vi "Zoom(User Event).vi"(8 "error in (no error)":errorcluster, 10 "Zoom":bool, 11 "XYGraphOverview in":refnum<class "XYGraphOverview.lvclass">) -> (0 "error out":errorcluster, 3 "XYGraphOverview out":refnum<class "XYGraphOverview.lvclass">)   [LabVIEW 2020, in "XYGraphOverview.lvlib" / "XYGraphOverview.lvclass"]
uses:
  XYGraphOverview.lvclass
  XYGraphOverview.lvclass/XYGraphOverview.ctl
  Read Block Color.vi
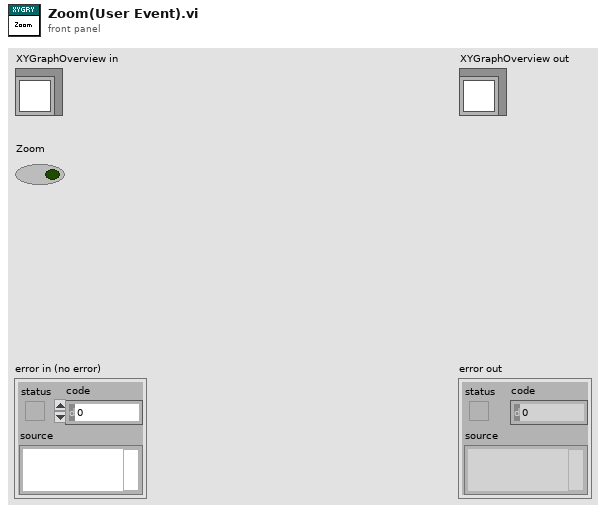
[diagram p1: front panel]
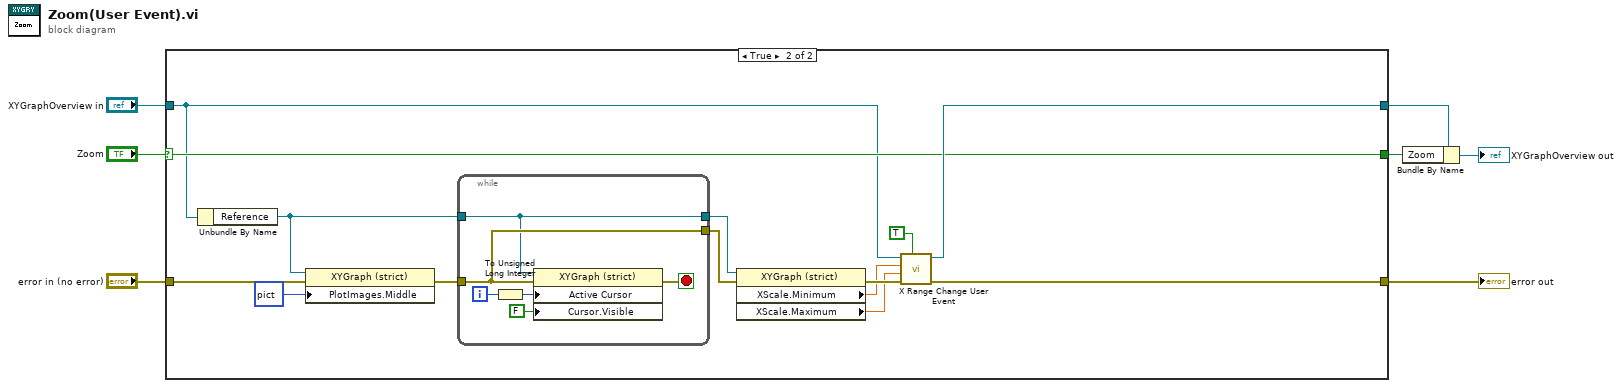
[diagram p0: block diagram]
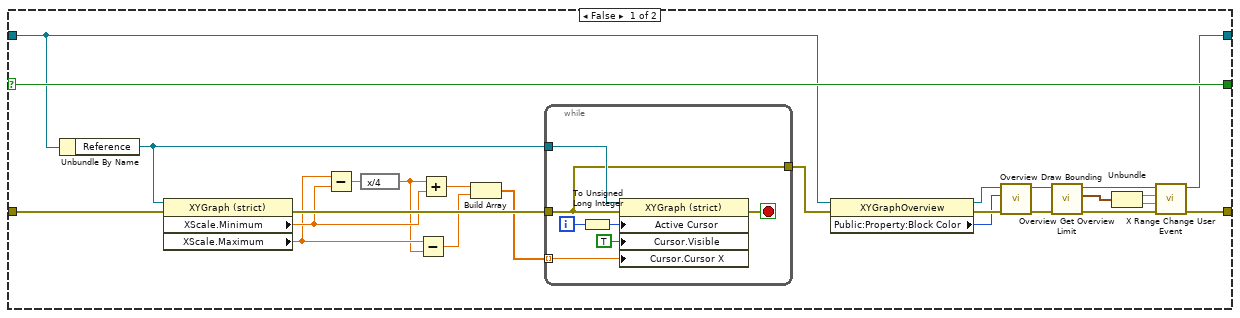
[diagram p2: hidden frame]
diagram:
  n1 = case shown="True" "Zoom" {
    selector: "Zoom" -> [w22 w46]
    tunnel: "error in (no error)" -> [w32 w52]
    tunnel: "XYGraphOverview in" -> [w9 w44]
    tunnel: [w8 w47] -> w3
    tunnel: [w10 w49] -> w7
    tunnel: [w22 w46] -> w2
    frame False {
      n2 = Unbundle By Name(w9) -> ("Reference"=w30:refnum<vi>)
      n3 = property class="XYGraph (strict)"(reference=w30, error in=w32) -> (error out=w31:errorcluster, "XScale.Minimum"=w28:dbl, "XScale.Maximum"=w27:dbl)  [unwired: 1 out]
      n4 = Subtract(x=w27, y=w28) -> (x-y=w29:dbl)
      n5 = expression code="x/4"(w29) -> (w26:dbl)
      n6 = Subtract(x=w27, y=w26) -> (x-y=w24:dbl)
      n7 = Add(x=w26, y=w28) -> (x+y=w25:dbl)
      n8 = Build Array(w25, w24) -> (w23:dbl[])
      n9 = while {
        tunnel: w31 -> [w34]
        tunnel: w30 -> [w35]
        tunnel: [w34] -> w11
        tunnel: w23 -> [w33] mode=indexing
        i -> [w38]
        stop <- w36 stop-if-true
        n10 = To Unsigned Long Integer(number=w38) -> (unsigned 32bit integer=w37:u32)
        n11 = property on="Property Node" class="XYGraph (strict)"(reference=w35, error in=w34, "Active Cursor"=w37, "Cursor.Visible"=TRUE, "Cursor.Cursor X"=w33) -> (error out=w36:errorcluster)  [unwired: 1 out]
      }
      n12 = property class="XYGraphOverview"(reference=w9, error in=w11) -> (reference out=w13:refnum<class "XYGraphOverview.lvclass">, error out=w14:errorcluster, "Public:Property:Block Color"=w12:u32)
      n13 = call "Overview Draw Bounding.vi"("error in (no error)"=w14, "Color"=w12, "XYGraphOverview in"=w13) -> ("error out"=w21:errorcluster, "XYGraphOverview out"=w20:refnum<class "XYGraphOverview.lvclass">)  [unwired: 7 in]
      n14 = call "Overview Get Overview Limit.vi"("error in"=w21, "XYGraphOverview in"=w20) -> ("error out"=w17:errorcluster, "Limit"=w19:cluster{"Lower Limit":dbl, "Upper Limit":dbl}, "XYGraphOverview out"=w18:refnum<class "XYGraphOverview.lvclass">)  [unwired: 7 in]
      n15 = Unbundle(w19) -> ("Lower Limit"=w16:dbl, "Upper Limit"=w15:dbl)
      n16 = call "X Range Change User Event.vi"("error in (no error)"=w17, "Upper Range"=w15, "Lower Range"=w16, "XYGraphOverview in"=w18) -> ("error out"=w10:errorcluster, "XYGraphOverview out"=w8:refnum<class "XYGraphOverview.lvclass">)  [unwired: 6 in]
    }
    frame True {
      n17 = Unbundle By Name(w44) -> ("Reference"=w50:refnum<vi>)
      n18 = property on="Property Node" class="XYGraph (strict)"(reference=w50, error in=w52, "PlotImages.Middle"=picture data[5B] ("Plot Images:Middle")) -> (error out=w51:errorcluster)  [unwired: 1 out]
      n19 = while {
        tunnel: w51 -> [w55]
        tunnel: w50 -> [w54]
        tunnel: [w55] -> w40
        tunnel: [w54] -> w45
        i -> [w58]
        stop <- w56 stop-if-true
        n20 = To Unsigned Long Integer(number=w58) -> (unsigned 32bit integer=w57:u32)
        n21 = property on="Property Node" class="XYGraph (strict)"(reference=w54, error in=w55, "Active Cursor"=w57, "Cursor.Visible"=FALSE) -> (error out=w56:errorcluster)  [unwired: 1 out]
      }
      n22 = property on="Property Node" class="XYGraph (strict)"(reference=w45, error in=w40) -> (error out=w43:errorcluster, "XScale.Minimum"=w42:dbl, "XScale.Maximum"=w41:dbl)  [unwired: 1 out]
      n23 = call "X Range Change User Event.vi"("All"=TRUE, "error in (no error)"=w43, "Upper Range"=w41, "Lower Range"=w42, "XYGraphOverview in"=w44) -> ("error out"=w49:errorcluster, "XYGraphOverview out"=w47:refnum<class "XYGraphOverview.lvclass">)  [unwired: 5 in]
    }
  }
  "error out" <- w7
  n24 = Bundle By Name(cluster=w3, "Zoom"=w2) -> (→"XYGraphOverview out":refnum<class "XYGraphOverview.lvclass">)
